vi "RS_gen_ON_OFF.vi"(0 "Generator Output":bool=TRUE, 2 "error in (no error)":errorcluster) -> (1 "error out":errorcluster)   [LabVIEW 2013]
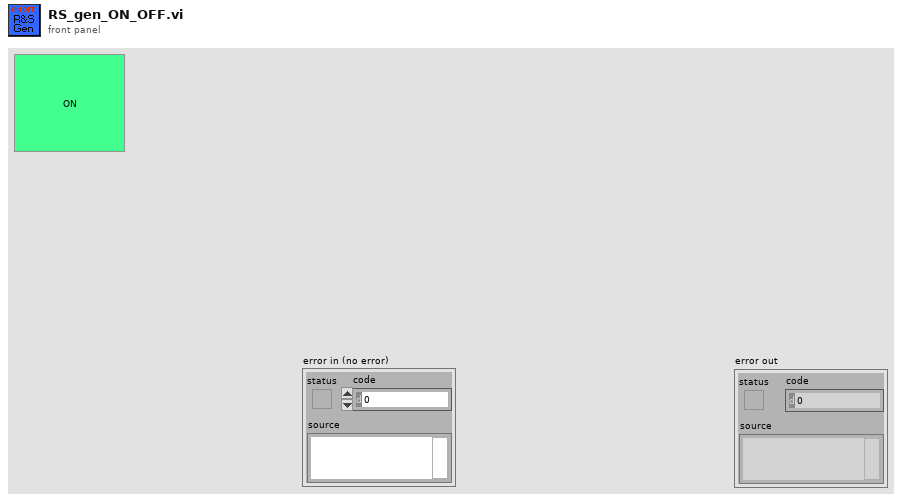
[diagram p1: front panel]
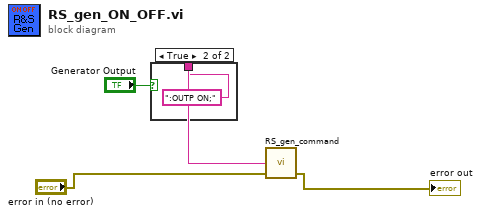
[diagram p0: block diagram]
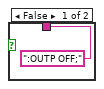
[diagram p2: hidden frame]
diagram:
  n1 = case shown="True" "Generator Output" {
    tunnel: [":OUTP OFF;" ":OUTP ON;"] -> w3
    frame False {
    }
    frame True {
    }
  }
  n2 = call "RS_gen_command.vi"("error in (no error)"="error in (no error)", "Comand"=w3) -> ("error out"=→"error out":errorcluster)  [unwired: 3 in]
